vi "Generate Simulated Data.vi"(8 "error in (no error)":errorcluster, 10 "DAQmx Task Name":refnum<k21>, 11 "Signal Type":T1=enum."Sine Wave") -> (0 "error out":errorcluster, 2 "Graph Data":waveform(dbl)[](array[waveform]))   [LabVIEW 2023, in "Acquisition.lvlib"]
doc: "Generates sample waveforms according to the signal type in the HW Config input."
uses:
  Acquisition.lvlib
  Signal Type.ctl
  <vilib>/DAQmx/read.llb/DAQmx Read (Analog 1D Wfm NChan 1Samp).vi
  <vilib>/DAQmx/miscellaneous.llb/DAQmx Fill In Error Info.vi
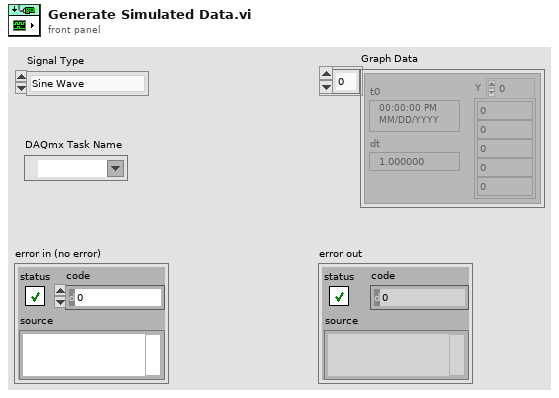
[diagram p1: front panel]
types:
  T1 = typedef "Acquisition.lvlib/Signal Type.ctl" = enum16{"Temperature", "Sine Wave", "Square with Noise"}
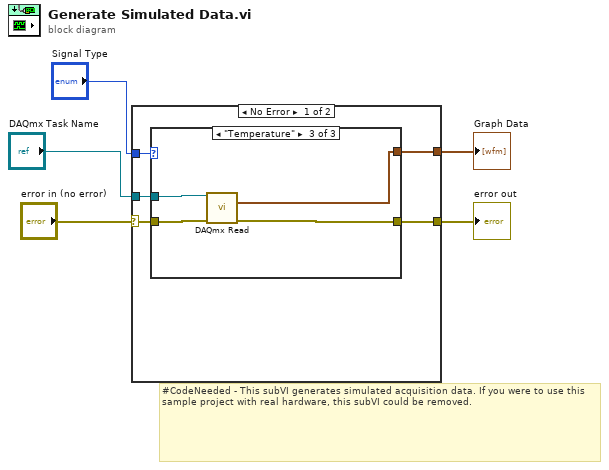
[diagram p0: block diagram]
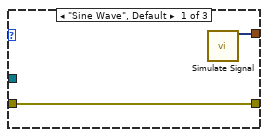
[diagram p2: hidden frame]
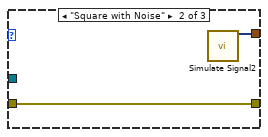
[diagram p3: hidden frame]
diagram:
  # "#CodeNeeded - This subVI generates simulated acquisition data. If you were to use this sample project with real hardware, this subVI could be removed."
  n1 = case shown="No Error" "error in (no error)" {
    selector: "error in (no error)" -> [w7 w19]
    tunnel: [w6 w19] -> w4
    tunnel: [w10 _] -> w3
    tunnel: "Signal Type" -> [w9 _]
    tunnel: "DAQmx Task Name" -> [w8 _]
    frame No Error {
      n2 = case shown="\"Temperature\"" w9 {
        tunnel: [w12 w14 w17] -> w10
        tunnel: w8 -> [_ _ w15]
        tunnel: w7 -> [w11 w13 w16]
        tunnel: [w11 w13 w18] -> w6
        frame "Sine Wave", Default {
          n3 = call "Simulate Signal"() -> ("Sine"=w12:dynamicdata)  [unwired: 14 in, 1 out]
        }
        frame "Square with Noise" {
          n4 = call "Simulate Signal2"() -> ("Square with Gaussian Noise"=w14:dynamicdata)  [unwired: 14 in, 1 out]
        }
        frame "Temperature" {
          n5 = call-poly <vilib>:"DAQmx Read.vi"("task/channels in"=w15, "error in"=w16) -> ("data"=w17:waveform(dbl)[], "error out"=w18:errorcluster)  [unwired: 11 in, 1 out]
        }
      }
    }
    frame Error {
    }
  }
  "error out" <- w4
  "Graph Data" <- w3
